vi "Notfi_Clean.vi"(8 "error in (no error)":errorcluster, 11 "NotifyIcon in":refnum<class "NotifyIcon.lvclass">) -> (0 "error out":errorcluster, 3 "NotifyIcon out":refnum<class "NotifyIcon.lvclass">)   [LabVIEW 2016, in "NotifyIcon.lvclass"]
uses:
  NotifyIcon.lvclass
  NotifyIcon.lvclass/NotifyIcon.ctl
  System.Windows.Forms
  ContexMenue/ContexMenue.lvclass
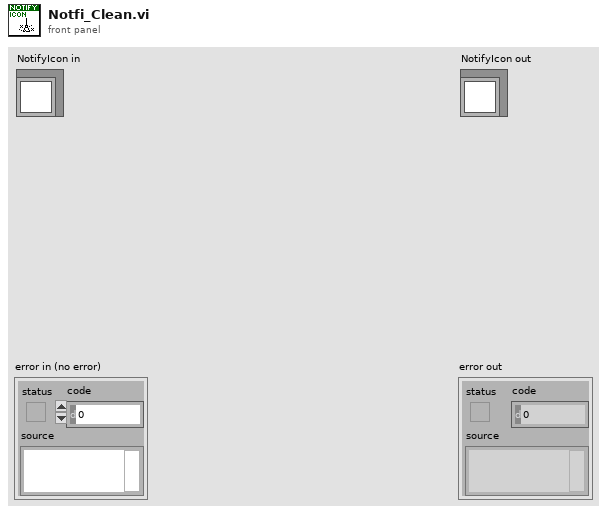
[diagram p1: front panel]
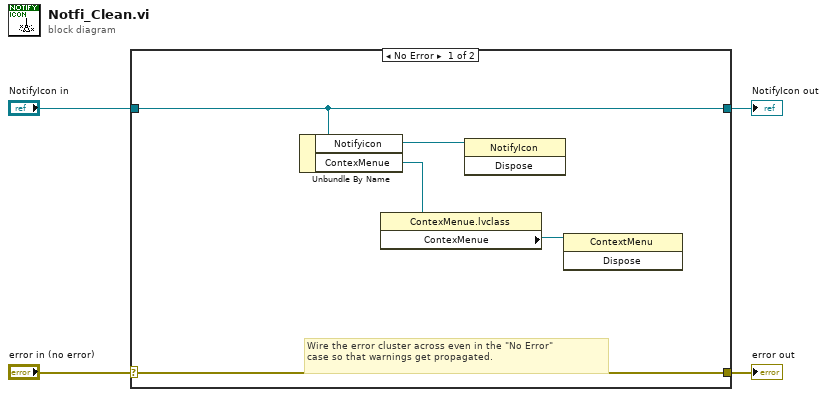
[diagram p0: block diagram]
diagram:
  n1 = case shown="No Error" "error in (no error)" {
    selector: "error in (no error)" -> [w9 w11]
    tunnel: [w9 w11] -> w3
    tunnel: [w8 w10] -> w1
    tunnel: "NotifyIcon in" -> [w8 w10]
    frame No Error {
      # "Wire the error cluster across even in the \"No Error\"\ncase so that warnings get propagated."
      n2 = Unbundle By Name(w8) -> ("Notifyicon"=w7:refnum<k24>, "ContexMenue"=w6:refnum<class "ContexMenue.lvclass">)
      n3 = property class="ContexMenue.lvclass"(reference=w6) -> ("ContexMenue"=w5:refnum<k24>)  [unwired: 1 in, 2 out]
      n4 = invoke class="NotifyIcon" method="Dispose"(reference=w7) -> ()  [unwired: 2 in, 3 out]
      n5 = invoke class="ContextMenu" method="Dispose"(reference=w5) -> ()  [unwired: 2 in, 3 out]
    }
    frame Error {
    }
  }
  "error out" <- w3
  "NotifyIcon out" <- w1
